vi "EvaluateFitCurves.vi"(0 "Zref":dbl=508.0 min=0.0, 1 "Fit Zmax":dbl, 2 "nPoints":i32, 3 "Fit Zmin":dbl, 5 "PowerLaw":T1) -> (6 "PlotCluster":cluster{"Array":dbl[], "Array":dbl[]})   [LabVIEW 2021]
uses:
  PowerLaw.ctl
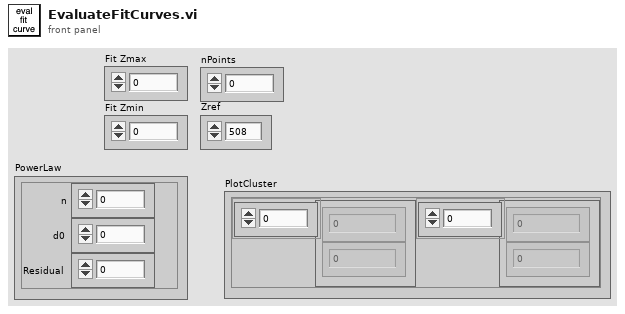
[diagram p1: front panel]
types:
  T1 = typedef "PowerLaw.ctl" = cluster{"n":dbl, "d0":dbl, "Residual":dbl}
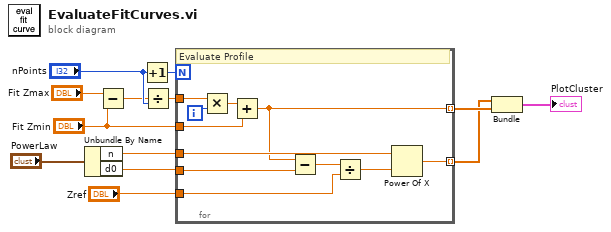
[diagram p0: block diagram]
diagram:
  n1 = Unbundle By Name("PowerLaw") -> ("n"=w7:dbl, "d0"=w6:dbl)
  n2 = Subtract(x="Fit Zmax", y="Fit Zmin") -> (x-y=w4:dbl)
  n3 = Increment(x="nPoints") -> (x+1=w1:i32)
  n4 = Divide(x=w4, y="nPoints") -> (x/y=w9:dbl)
  n5 = for {
    N: w1 -> [_]
    tunnel: w9 -> [w24]
    tunnel: [w15] -> w12 mode=indexing
    tunnel: w6 -> [w21]
    tunnel: w7 -> [w20]
    tunnel: [w17] -> w11 mode=indexing
    tunnel: "Zref" -> [w16]
    tunnel: "Fit Zmin" -> [w14]
    i -> [w23]
    # "Evaluate Profile"
    n6 = Multiply(x=w24, y=w23) -> (x*y=w22:dbl)
    n7 = Add(x=w22, y=w14) -> (x+y=w15:dbl)
    n8 = Subtract(x=w15, y=w21) -> (x-y=w19:dbl)
    n9 = Divide(x=w19, y=w16) -> (x/y=w18:dbl)
    n10 = Power Of X(1:w18, 2:w20) -> (0:w17:dbl)
  }
  n11 = Bundle(w11, w12) -> (→"PlotCluster":cluster{dbl[], dbl[]})  [unwired: 1 in]
